vi "K2000_read_meas-register.vi"(2 "error out 2":errorcluster, 4 "GPIB Address":string) -> (0 "error out":errorcluster, 1 "Boolean":bool)   [LabVIEW 2013]
panel:
  out "data":string
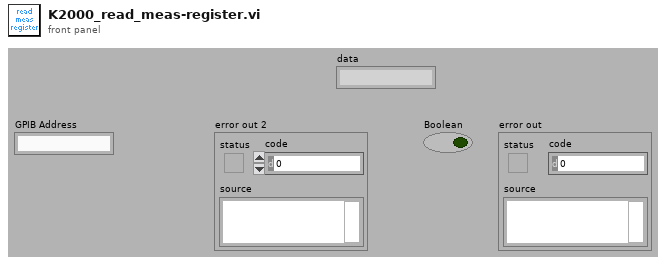
[diagram p1: front panel]
types:
  T1 = enum16{"big-endian, network order", "native, host order", "little-endian"}
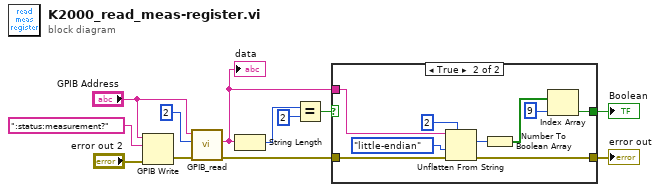
[diagram p0: block diagram]
diagram:
  n1 = GPIB Write(0:"GPIB Address", 1:":status:measurement?" ("data"), 3:"error out 2") -> (6:w4:errorcluster)  [unwired: 3 out]
  n2 = call "GPIB_read.vi"("error out 2"=w4, "bytes"=2, "GPIB Address"="GPIB Address") -> ("error out"=w10:errorcluster, "data"=w6:string)  [unwired: 7 out]
  "data" <- w6
  n3 = String Length(string=w6) -> (length=w2:i32)
  n4 = Equal?(x=w2, y=2) -> (x = y?=w7:bool)
  n5 = case shown="True" w7 {
    selector: w7 -> [w14 _]
    tunnel: w6 -> [_ w21]
    tunnel: [w14 w18] -> w12
    tunnel: w10 -> [w13 w16]
    tunnel: [w13 w15] -> w11
    frame False {
    }
    frame True {
      n6 = Unflatten From String(type=u16 2 ("bytes"), binary string=w21, byte order (0:big-endian, network order)=T1."little-endian", error in (no error)=w16) -> (value=w22:u16, error out=w15:errorcluster)  [unwired: 2 out]
      n7 = Number To Boolean Array(number=w22) -> (Boolean array=w20:bool[])
      n8 = Index Array(array=w20, index=9) -> (element=w18:bool)
    }
  }
  "Boolean" <- w12
  "error out" <- w11
